vi "Servos.vi"() -> ()   [LabVIEW 2019]
uses:
  <vilib>/myRIO/Instrument Drivers/Onboard IO/PWM/typedefs/PWM Reference.ctl
  <vilib>/myRIO/Common/Instrument Driver Framework/Utilities/typedefs/myRIO Generic Hardware Reference.ctl
  <vilib>/myRIO/Common/Instrument Driver Framework/Utilities/typedefs/Hardware Version Enum.ctl
  <vilib>/myRIO/Common/Instrument Driver Framework/Utilities/typedefs/myRIO v1.0 Reference.ctl
  <vilib>/myRIO/Common/Instrument Driver Framework/Utilities/typedefs/Generic FPGA Reference.ctl
  <vilib>/myRIO/Common/Instrument Driver Framework/myRIO v1.0/PWM/typedefs/PWM Channels Enum.ctl
  <vilib>/myRIO/Instrument Drivers/Onboard IO/PWM/typedefs/PWM Configuration.ctl
  <vilib>/userdefined/High Color/nirio_resource_hc.ctl
  <vilib>/myRIO/Common/Instrument Driver Framework/Utilities/vis/Is FPGA Ref Available.vi
  <vilib>/myRIO/Common/Instrument Driver Framework/myRIO v1.0/PWM/vis/myRIO v1.1 Open PWM.vi
  <vilib>/myRIO/Instrument Drivers/Onboard IO/PWM/vis/Set Duty Cycle and Frequency.vi
  <vilib>/myRIO/Common/Instrument Driver Framework/Utilities/vis/Validate Channels.vi
  <vilib>/myRIO/Common/Instrument Driver Framework/myRIO v1.0/PWM/vis/myRIO v1.0 Reserve PWM.vi
  <vilib>/myRIO/Common/Instrument Driver Framework/myRIO v1.0/PWM/vis/myRIO v1.0 Build MUX Configuration PWM.vi
  <vilib>/myRIO/Common/Instrument Driver Framework/myRIO v1.0/Resource Manager/vis/myRIO v1.0 Reserve Channel List.vi
  <vilib>/myRIO/Common/Instrument Driver Framework/myRIO v1.0/Resource Manager/vis/myRIO v1.0 Create Configuration List.vi
  <vilib>/myRIO/Common/Instrument Driver Framework/myRIO v1.0/Resource Manager/vis/myRIO v1.0 Reserve Channel.vi
  <vilib>/myRIO/Common/Instrument Driver Framework/myRIO v1.0/Resource Manager/vis/myRIO v1.0 Unreserve Channel.vi
  <vilib>/myRIO/Common/Instrument Driver Framework/myRIO v1.0/Resource Manager/vis/myRIO v1.0 Build Mutex Name.vi
  <vilib>/Utility/VariantDataType/GetNumericInfo.vi
  <vilib>/Utility/error.llb/Error Cluster From Error Code.vi
  <vilib>/myRIO/Common/Instrument Driver Framework/myRIO v1.0/myRIO v1.1 Open.vi
  <vilib>/myRIO/Common/Instrument Driver Framework/Utilities/vis/IO Manager.vi
  <vilib>/myRIO/Common/Instrument Driver Framework/Utilities/vis/Configuration Manager.vi
  <vilib>/myRIO/Common/Instrument Driver Framework/myRIO v1.0/Resource Manager/vis/myRIO v1.0 Configure IO.vi
  <vilib>/myRIO/Common/Instrument Driver Framework/myRIO v1.0/myRIO v1.0 Close.vi
  <vilib>/myRIO/Common/Instrument Driver Framework/myRIO v1.0/PWM/vis/myRIO v1.0 Write PWM.vi
  <vilib>/myRIO/Express VI/Onboard IO/PWM/PWM Express VI.xnode
  <vilib>/myRIO/Instrument Drivers/Onboard IO/PWM/vis/myRIO PWM Open.xnode
  <vilib>/myRIO/Instrument Drivers/Onboard IO/PWM/PWM.lvlib
panel:
  out "y":dbl
  out "x":dbl
  out "Duty tilt":dbl format="%#_13g"
  out "Duty pan":dbl format="%#_13g"
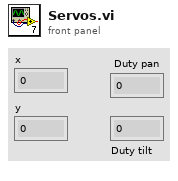
[diagram p1: front panel]
types:
  T1 = typedef "PWM.lvlib/PWM Reference.ctl" = cluster{"myRIO Reference":T2, "PWM Channels Enum":T6, "PWM Configuration":T7}
  T2 = typedef "myRIO Generic Hardware Reference.ctl" = cluster{"myRIO Model":T3, "myRIO Hardware Reference":T4}
  T3 = typedef "Hardware Version Enum.ctl" = enum16{"Unknown", "myRIO-1900", "myRIO-1950", "roboRIO", "NI ELVIS RIO CM", "ELVIS III"}
  T4 = typedef "myRIO v1.0 Reference.ctl" = cluster{"Generic FPGA Reference":T5, "Allow multiple opens":bool}
  T5 = typedef "Generic FPGA Reference.ctl" = refnum<k20>
  T6 = typedef "PWM Channels Enum.ctl" = enum16{"Not Connected", "C/PWM0", "C/PWM1", "A/PWM0", "A/PWM1", "A/PWM2", "A/PWM3", "A/PWM4", "A/PWM5", "A/PWM6", "A/PWM7", "A/PWM8", "A/PWM9", "A/PWM10", "A/PWM11", "A/PWM12", "A/PWM13", "A/PWM14", "A/PWM15", "A/PWM16", "A/PWM17", "A/PWM18", "A/PWM19", "B/PWM0", "B/PWM1", "B/PWM2", "B/PWM3", "B/PWM4", "B/PWM5", "B/PWM6", "B/PWM7", "B/PWM8", "B/PWM9", "B/PWM10", "B/PWM11", "B/PWM12", "B/PWM13", "B/PWM14", "B/PWM15", "B/PWM16", "B/PWM17", "B/PWM18", "B/PWM19", "PWM/PWM0", "PWM/PWM1", "PWM/PWM2", "PWM/PWM3", "PWM/PWM4", "PWM/PWM5", "PWM/PWM6", "PWM/PWM7", "PWM/PWM8", "PWM/PWM9"}
  T7 = typedef "PWM.lvlib/PWM Configuration.ctl" = cluster{"Frequency":dbl, "Duty Cycle":dbl}
  T8 = typedef "nirio_resource_hc.ctl" = tag
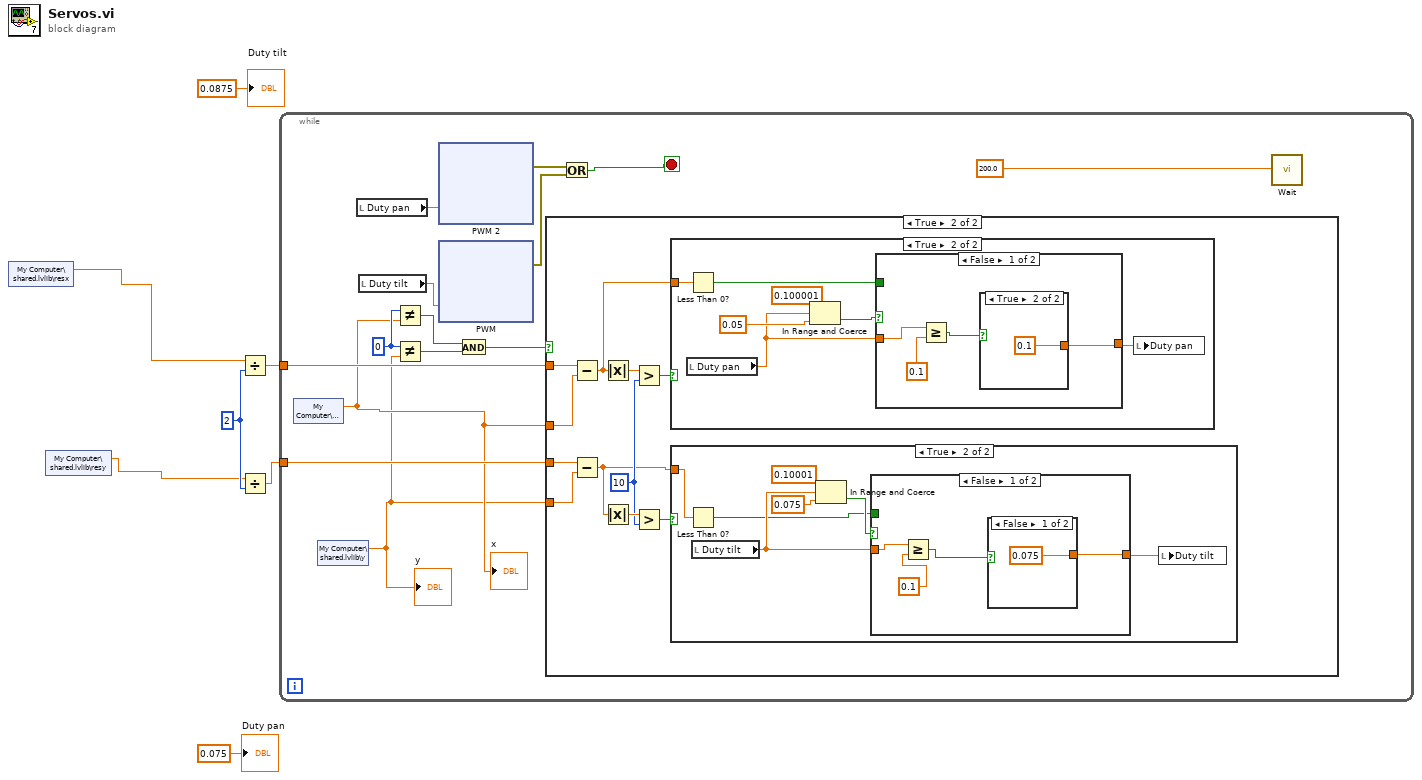
[diagram p0: block diagram]
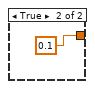
[diagram p4: hidden frame]
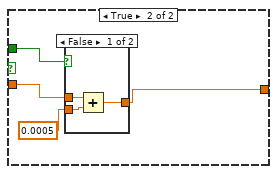
[diagram p5: hidden frame]
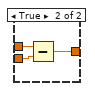
[diagram p6: hidden frame]
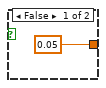
[diagram p8: hidden frame]
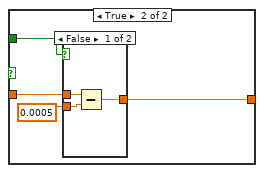
[diagram p9: hidden frame]
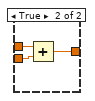
[diagram p10: hidden frame]
diagram:
  w7 = 2
  n1 = shared-variable "My Computer\\shared.lvlib\\resx"() -> (w1:dbl)  [unwired: 1 in, 1 out]
  n2 = shared-variable "My Computer\\shared.lvlib\\resy"() -> (w2:dbl)  [unwired: 1 in, 1 out]
  n3 = Divide(x=w1, y=w7) -> (x/y=w6:dbl)
  n4 = Divide(x=w2, y=w7) -> (x/y=w5:dbl)
  n5 = while {
    tunnel: w6 -> [w17]
    tunnel: w5 -> [w16]
    stop <- w11 stop-if-true
    w21 = 0
    n6 = shared-variable "My Computer\\shared.lvlib\\x"() -> (w10:dbl)  [unwired: 1 in, 1 out]
    "x" <- w10
    n7 = shared-variable "My Computer\\shared.lvlib\\y"() -> (w9:dbl)  [unwired: 1 in, 1 out]
    "y" <- w9
    n8 = local read "Duty pan"() -> (w14:dbl)
    n9 = local read "Duty tilt"() -> (w15:dbl)
    n10 = Not Equal?(x=w21, y=w10) -> (x != y?=w20:bool)
    n11 = Not Equal?(x=w21, y=w9) -> (x != y?=w19:bool)
    n12 = xnode "PWM 2"("Duty Cycle"=w14) -> ("error out"=w12:errorcluster)  [unwired: 1 in]
    n13 = xnode "PWM"("Duty Cycle"=w15) -> ("error out"=w13:errorcluster)  [unwired: 1 in]
    n14 = And(x=w20, y=w19) -> (x .and. y?=w18:bool)
    n15 = case shown="True" w18 {
      tunnel: w9 -> [_ w27]
      tunnel: w10 -> [_ w31]
      tunnel: w17 -> [_ w32]
      tunnel: w16 -> [_ w29]
      frame False {
      }
      frame True {
        w26 = 10
        n16 = Subtract(x=w32, y=w31) -> (x-y=w22:dbl)
        n17 = Subtract(x=w29, y=w27) -> (x-y=w23:dbl)
        n18 = Absolute Value(x=w22) -> (abs(x)=w30:dbl)
        n19 = Absolute Value(x=w23) -> (abs(x)=w28:dbl)
        n20 = Greater?(x=w30, y=w26) -> (0:w25:bool)
        n21 = Greater?(x=w28, y=w26) -> (0:w24:bool)
        n22 = case shown="True" w25 {
          tunnel: w22 -> [_ w62]
          frame False {
          }
          frame True {
            n23 = local read "Duty pan"() -> (w59:dbl)
            n24 = Less Than 0?(x=w62) -> (x < 0?=w56:bool)
            n25 = In Range and Coerce(upper limit=0.100001, x=w59, lower limit=0.05) -> (In Range?=w57:bool)  [unwired: 1 out]
            n26 = case shown="False" w57 {
              tunnel: w59 -> [w66 w72]
              tunnel: [w63 w70] -> w58
              tunnel: w56 -> [_ w69]
              frame False {
                n27 = Greater Or Equal?(x=w66, y=0.1) -> (x >= y?=w64:bool)
                n28 = case shown="True" w64 {
                  tunnel: [0.05 0.1] -> w63
                  frame False {
                  }
                  frame True {
                  }
                }
              }
              frame True {
                n29 = case shown="False" w69 {
                  tunnel: w72 -> [w75 w78]
                  tunnel: 0.0005 -> [w74 w77]
                  tunnel: [w73 w76] -> w70
                  frame False {
                    n30 = Subtract(x=w75, y=w74) -> (x-y=w73:dbl)
                  }
                  frame True {
                    n31 = Add(x=w78, y=w77) -> (x+y=w76:dbl)
                  }
                }
              }
            }
            n32 = local write "Duty pan"(w58) -> ()
          }
        }
        n33 = case shown="True" w24 {
          tunnel: w23 -> [_ w39]
          frame False {
          }
          frame True {
            n34 = Less Than 0?(x=w39) -> (x < 0?=w33:bool)
            n35 = local read "Duty tilt"() -> (w36:dbl)
            n36 = In Range and Coerce(upper limit=0.10001, x=w36, lower limit=0.075) -> (In Range?=w34:bool)  [unwired: 1 out]
            n37 = case shown="False" w34 {
              tunnel: w36 -> [w43 w49]
              tunnel: [w40 w47] -> w35
              tunnel: w33 -> [_ w46]
              frame False {
                n38 = Greater Or Equal?(x=w43, y=0.1) -> (x >= y?=w41:bool)
                n39 = case shown="False" w41 {
                  tunnel: [0.075 0.1] -> w40
                  frame False {
                  }
                  frame True {
                  }
                }
              }
              frame True {
                n40 = case shown="False" w46 {
                  tunnel: w49 -> [w52 w55]
                  tunnel: 0.0005 -> [w51 w54]
                  tunnel: [w50 w53] -> w47
                  frame False {
                    n41 = Add(x=w52, y=w51) -> (x+y=w50:dbl)
                  }
                  frame True {
                    n42 = Subtract(x=w55, y=w54) -> (x-y=w53:dbl)
                  }
                }
              }
            }
            n43 = local write "Duty tilt"(w35) -> ()
          }
        }
      }
    }
    n44 = Or(x=w12, y=w13) -> (x .or. y?=w11:bool)
    n45 = call "Wait"("Count(mSec)"=200.0) -> ()  [unwired: 1 out]
  }
  "Duty pan" <- 0.075
  "Duty tilt" <- 0.0875
